vi "Workspace Map.vi"(11 "Assembly Tray Region":i32) -> (2 "Pick Up Tool Region":i32, 3 "Component Tray Region":i32)   [LabVIEW 2020, in "Fixture.lvclass"]
uses:
  Fixture.lvclass
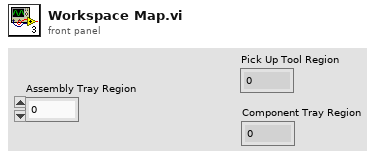
[diagram p1: front panel]
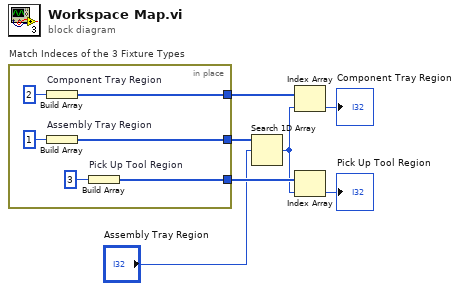
[diagram p0: block diagram]
diagram:
  n1 = in-place "Match Indeces of the 3 Fixture Types" {
    in-place-border: [w11] -> w7
    in-place-border: [w10] -> w5
    in-place-border: [w8] -> w3
    n2 = Build Array "Component Tray Region"(2) -> (w11:i32[])
    n3 = Build Array "Assembly Tray Region"(1) -> (w8:i32[])
    n4 = Build Array "Pick Up Tool Region"(3) -> (w10:i32[])
  }
  n5 = Search 1D Array(1D array=w3, element="Assembly Tray Region") -> (index of element=w1:i32)  [unwired: 1 in]
  n6 = Index Array(array=w7, index=w1) -> (element=→"Component Tray Region":i32)
  n7 = Index Array(array=w5, index=w1) -> (element=→"Pick Up Tool Region":i32)
